vi "prb1.vi"() -> ()   [LabVIEW 2017]
panel:
  in  "STOP":bool
  out "LED":bool
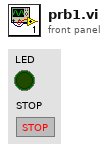
[diagram p1: front panel]
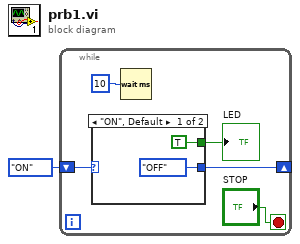
[diagram p0: block diagram]
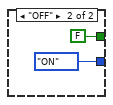
[diagram p2: hidden frame]
diagram:
  n1 = while {
    shift-right: [w5] -> _
    shift-left: enum16{"ON", "OFF"}."ON" -> [w6]
    stop <- "STOP" stop-if-true
    n2 = case shown="\"ON\", Default" w6 {
      tunnel: [enum16{"ON", "OFF", "STOP"}."OFF" enum16{"ON", "OFF"}."ON"] -> w5
      tunnel: [TRUE FALSE] -> w2
      frame "ON", Default {
      }
      frame "OFF" {
      }
    }
    "LED" <- w2
    n3 = Wait (ms)(milliseconds to wait=10) -> ()  [unwired: 1 out]
  }
